vi "Add Tool From VI.vi"(8 "error in (no error)":errorcluster, 10 "vi path":path, 11 "PyServer in":refnum<class "PyServer.lvclass">) -> (0 "error out":errorcluster, 3 "PyServer out":refnum<class "PyServer.lvclass">)   [LabVIEW 2025, in "Tools.lvlib"]
uses:
  Tools.lvlib
  PyServer/PyServer.lvclass
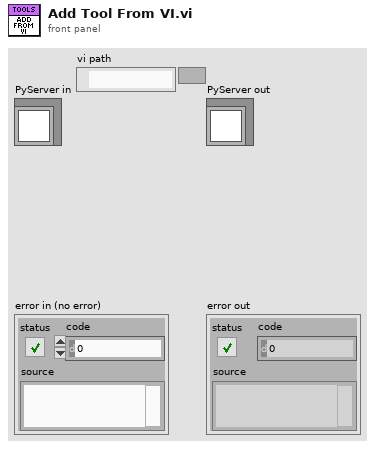
[diagram p1: front panel]
types:
  T1 = typedef "Tools.lvlib/Datatypes.ctl" = enum16{"Float", "Int", "String", "String Array", "Int Array", "Float Array", "Bool Array", "Bool", "Invalid"}
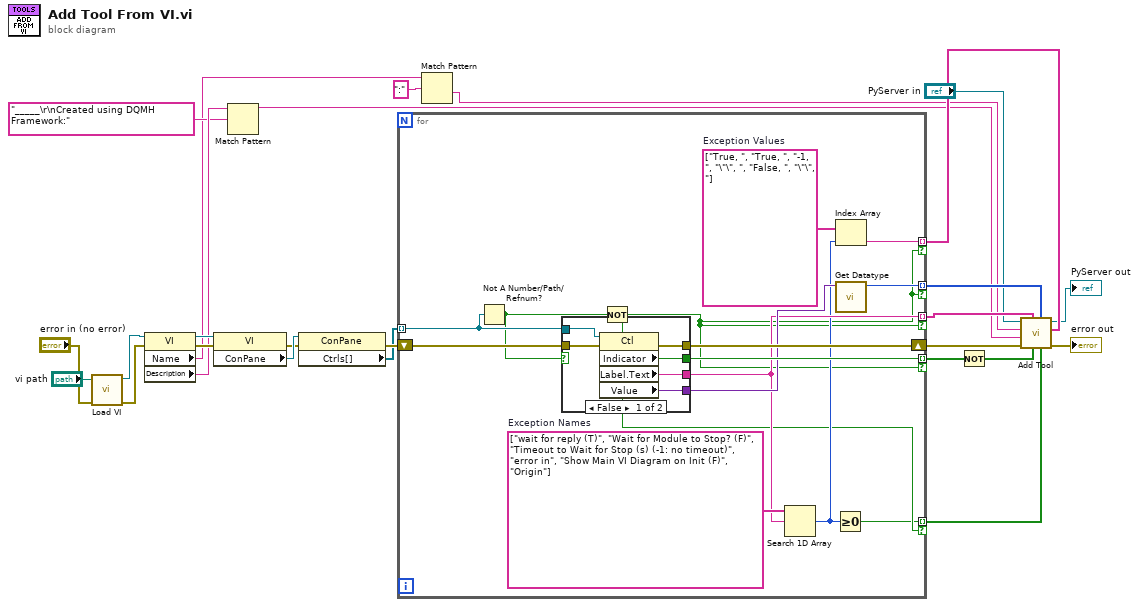
[diagram p0: block diagram]
diagram:
  n1 = call "Load VI.vi"("error in (no error)"="error in (no error)", "vi path"="vi path") -> ("error out"=w3:errorcluster, "VI out"=w2:refnum<vi>)  [unwired: 8 in]
  n2 = property class="VI"(reference=w2, error in=w3) -> (reference out=w16:refnum<vi>, error out=w17:errorcluster, "Name"=w8:string, "Description"=w12:string)
  n3 = property class="VI"(reference=w16, error in=w17) -> (error out=w14:errorcluster, "ConPane"=w15:refnum<vi>)  [unwired: 1 out]
  n4 = Match Pattern(string=w12, regular expression="_____\r\nCreated using DQMH Framework:") -> (before substring=w13:string)  [unwired: 1 in, 3 out]
  n5 = property class="ConPane"(reference=w15, error in=w14) -> (error out=w19:errorcluster, "Ctrls[]"=w18:refnum<vi>[])  [unwired: 1 out]
  n6 = for {
    tunnel: w18 -> [w40] mode=indexing
    shift-right: [w38] -> w20
    shift-left: w19 -> [w39]
    tunnel: [w37] -> w21 mode=indexing if=w28
    tunnel: [w32] -> w23 mode=indexing if=w28
    tunnel: [w36] -> w24 mode=indexing if=w28
    tunnel: [w31] -> w25 mode=indexing if=w28
    tunnel: [w27] -> w26 mode=indexing if=w28
    w34 = string[] ["True, ", "True, ", "-1, ", "\"\", ", "False, ", "\"\", "]  # Exception Values
    w33 = string[] ["wait for reply (T)", "Wait for Module to Stop? (F)", "Timeout to Wait for Stop (s) (-1: no timeout)", "error in", "Show Main VI Diagram on Init (F)", "Origin"]  # Exception Names
    n7 = Not A Number/Path/Refnum?(number/path/refnum=w40) -> (NaN/Path/Refnum?=w29:bool)
    n8 = case shown="False" w29 {
      tunnel: w40 -> [w46 _]
      tunnel: w39 -> [w45 w47]
      tunnel: [w44 w47] -> w38
      tunnel: [w43 _] -> w37
      tunnel: [w42 _] -> w35
      tunnel: [w41 _] -> w32
      frame False {
        n9 = property class="Ctl"(reference=w46, error in=w45) -> (error out=w44:errorcluster, "Indicator"=w43:bool, "Label.Text"=w41:string, "Value"=w42:variant)  [unwired: 1 out]
      }
      frame True {
      }
    }
    n10 = Not(x=w29) -> (.not. x?=w28:bool)
    n11 = Search 1D Array(1D array=w33, element=w32) -> (index of element=w30:i32)  [unwired: 1 in]
    n12 = Greater Or Equal To 0?(x=w30) -> (x >= 0?=w27:bool)
    n13 = Index Array(array=w34, index=w30) -> (element=w31:string)
    n14 = call "Get Datatype.vi"("Value"=w35) -> ("datatypes"=w36:T1)  [unwired: 10 in]
  }
  n15 = Match Pattern(string=w8, regular expression=":") -> (after substring=w10:string)  [unwired: 1 in, 3 out]
  n16 = Not(x=w21) -> (.not. x?=w22:bool[])
  n17 = call "Add Tool.vi"("Exception Values"=w25, "ignored?"=w26, "Parameter Types"=w24, "Input?"=w22, "Parameter Names"=w23, "error in (no error)"=w20, "Description"=w13, "Name"=w10, "PyServer in"="PyServer in") -> ("error out"=→"error out":errorcluster, "PyServer out"=→"PyServer out":refnum<class "PyServer.lvclass">)  [unwired: 1 in]
